vi "LV to ITX XY AutoPlot.vi"(4 "X,Y Log":i32[](array[numeric]), 6 "X,Y Labels":string[](array[string])=["x label", "y label"], 7 "Notes":string, 8 "error in":errorcluster, 10 "XY-Data []":cluster{"X  array":dbl[], "Y  Array":dbl[]}[](array[cluster]), 11 "path":path=path "C:/Users/voodoo.SEAGATE/Desktop/datatest") -> (0 "error out":errorcluster, 3 "file":path=path "C:/Users/voodoo.SEAGATE/Desktop/datatest/datatest.000019.itx")   [LabVIEW 2019, in "Data.ITX.lvclass"]
doc: "Write your XY data to ITX file. This AutoPlot VI adds commands to automatically create a graph in Igor to quickly view your data.\n\n-- path: base path to save data\n-- filename: base filename\n-- Notes: add any notes here to help you remember what experiment you did\n-- XY Array: Array of Clusters (ie, Array of XY graphs)\n-- wavenames: Give each data array a unique name such as \"time, bias, current,...\"\n-- X,Y Labels: For plotting in Igor. Can be ignored.\n-- X,Y Log: Do you wan to show X or Y on Log scale in Igor?"
uses:
  Data.ITX.lvclass
  Data/Data.lvclass
  Data/Typedefs/Operation--enum.ctl
panel:
  # "Below are relevant for creating graphs in Igor"
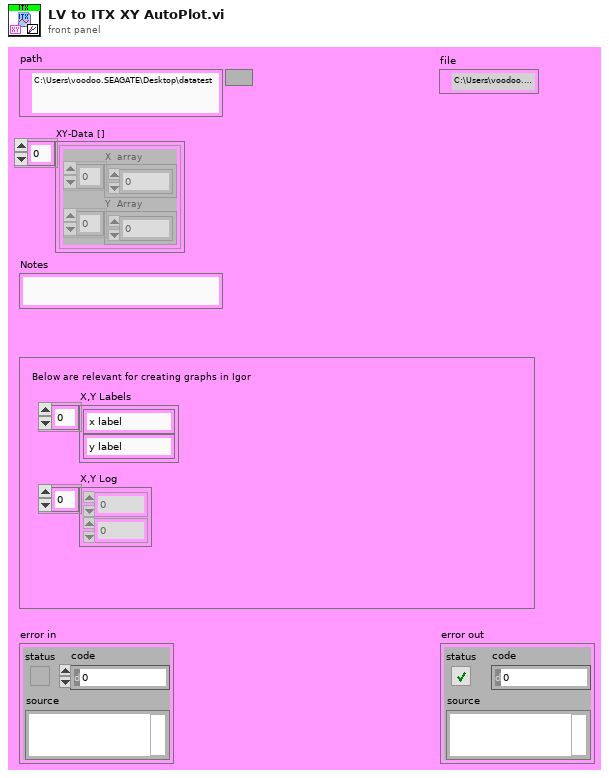
[diagram p1: front panel]
types:
  T1 = typedef "Data.lvclass/Operation--enum.ctl" = enum16{"Read", "Write", "Write + Append"}
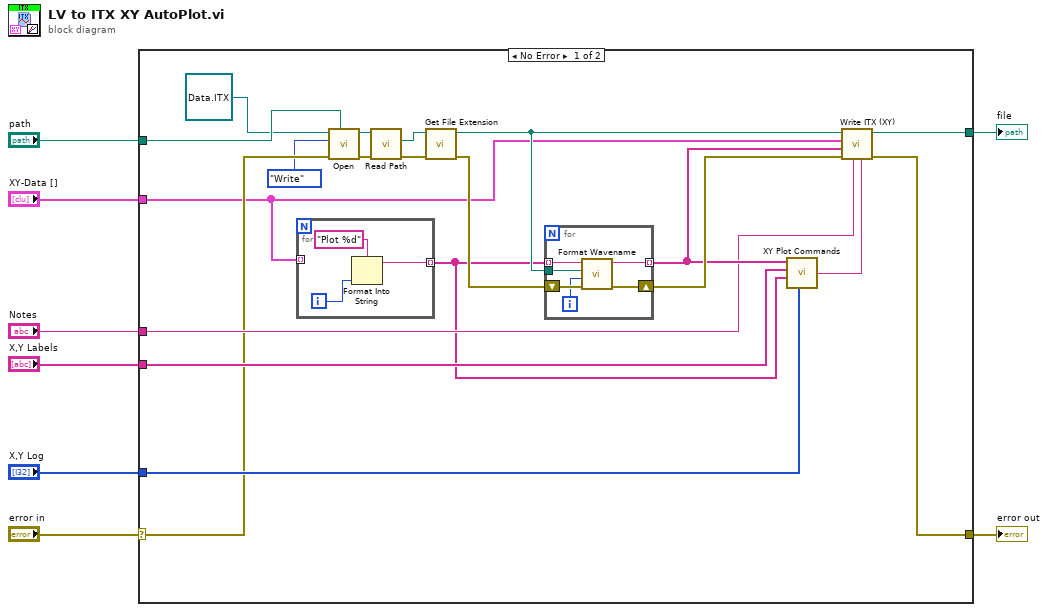
[diagram p0: block diagram]
diagram:
  n1 = case shown="No Error" "error in" {
    selector: "error in" -> [w12 w39]
    tunnel: "path" -> [w16 w38]
    tunnel: "X,Y Labels" -> [w28 _]
    tunnel: [w27 w38] -> w6
    tunnel: "X,Y Log" -> [w26 _]
    tunnel: "XY-Data []" -> [w10 _]
    tunnel: [w24 w39] -> w2
    tunnel: "Notes" -> [w21 _]
    frame No Error {
      n2 = for {
        tunnel: w10 -> [_] mode=indexing
        tunnel: [w29] -> w9 mode=indexing
        i -> [w31]
        n3 = Format Into String(format string="Plot %d", w31) -> (resulting string=w29:string)  [unwired: 2 in, 1 out]
      }
      n4 = call-dynamic "Open.vi"("Path"=w16, "error in (no error)"=w12, "Operation"=Operation--enum."Write", "Data in"=refnum<class "Data.ITX.lvclass"> refnum ("Data.ITX.lvclass")) -> ("error out"=w13:errorcluster, "Data out"=w14:refnum<class "Data.ITX.lvclass">)  [unwired: 6 in]
      n5 = call "Read Path.vi"("error in (no error)"=w13, "Data Save"=w14) -> ("error out"=w19:errorcluster, "Path"=w20:path)  [unwired: 7 in, 1 out]
      n6 = call <vilib>:"Get File Extension.vi"("error in (no error)"=w19, "file"=w20) -> ("error out"=w17:errorcluster, "dup file"=w18:path)  [unwired: 5 in, 3 out]
      n7 = for {
        tunnel: w9 -> [w37] mode=indexing
        shift-right: [w35] -> w25
        shift-left: w17 -> [w36]
        tunnel: [w34] -> w23 mode=indexing
        tunnel: w18 -> [w32]
        i -> [w33]
        n8 = call "Format Wavename.vi"("error in (no error)"=w36, "Index"=w33, "Path"=w32, "Name"=w37) -> ("error out"=w35:errorcluster, "Formatted wavename"=w34:string)  [unwired: 6 in]
      }
      n9 = call "XY Plot Commands.vi"("X,Y Log"=w26, "Plot labels"=w9, "X,Y Labels"=w28, "wavenames"=w23) -> ("result string"=w22:string)  [unwired: 2 in]
      n10 = call "Write ITX (XY).vi"("Commands"=w22, "Notes"=w21, "error in"=w25, "wavenames"=w23, "XY Array"=w10, "filename"=w18) -> ("error out"=w24:errorcluster, "file"=w27:path)  [unwired: 4 in]
    }
    frame Error {
    }
  }
  "file" <- w6
  "error out" <- w2
